vi "Reset Delay.vi"(2 "CIFCorePlugin in":refnum<class "CIFCorePlugin.lvclass">) -> (4 "Reset":bool)   [LabVIEW 2021, in "CIFCorePlugin.lvclass"]
doc: "Store a reset history for 2 cycles. This can be used for benchmarking where jitter may occur on startup or on reset/reinitialization."
uses:
  CIFCorePlugin.lvclass
  CIFCorePlugin.lvclass/CIFCorePlugin.ctl
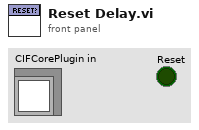
[diagram p1: front panel]
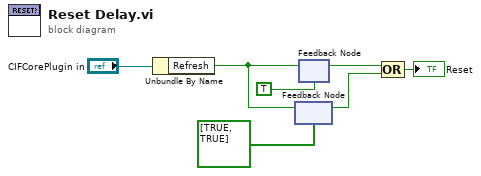
[diagram p0: block diagram]
diagram:
  n1 = Unbundle By Name("CIFCorePlugin in") -> ("Refresh"=w6:bool)
  n2 = feedback #1(bool[] [TRUE, TRUE]) -> (w3:bool)
  n3 = feedback-in #1(w6) -> ()
  n4 = feedback-in #2(w6) -> ()
  n5 = feedback #2(TRUE ("Refresh")) -> (w4:bool)
  n6 = Compound Arithmetic op=OR(w4, w3) -> (→"Reset":bool)
